vi "Set 2D CDB Q on Variant.vi"(8 "error in (no error)":errorcluster, 10 "2D CDB Data Q":T1, 11 "Variant in":variant) -> (0 "error out":errorcluster, 2 "replaced":bool, 3 "Variant out":variant)   [LabVIEW 2020, in "Internal Comm Classes.lvlib" / "WPL Comm (2D CDB).lvclass"]
uses:
  WPL Comm (2D CDB).lvclass
  Waveform 2d cdb queue.ctl
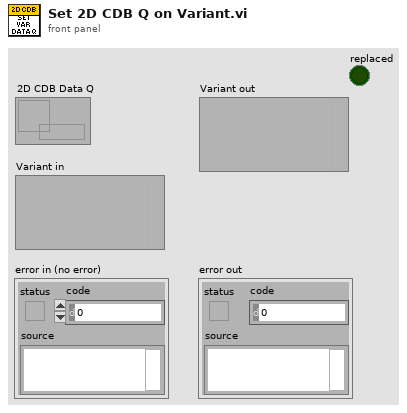
[diagram p1: front panel]
types:
  T1 = typedef "Internal Comm Classes.lvlib/WPL Comm (2D CDB).lvclass/Waveform 2d cdb queue.ctl" = refnum<queue>
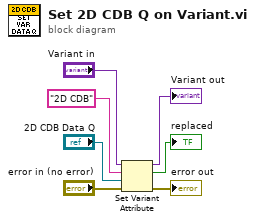
[diagram p0: block diagram]
diagram:
  n1 = Set Variant Attribute(Variant="Variant in", name="2D CDB", value="2D CDB Data Q", error in="error in (no error)") -> (Variant out=→"Variant out":variant, replaced=→"replaced":bool, error out=→"error out":errorcluster)
